vi "Broadcast Single Message.vi"(8 "error in (no error)":errorcluster, 9 "Mail Strategy In":refnum<class "Mail Strategy.lvclass">, 10 "Message In":refnum<class "Message.lvclass">, 11 "Map Tree Queue Messenger in":refnum<class "Map Tree Queue Messenger.lvclass">) -> (0 "error out":errorcluster, 3 "Map Tree Queue Messenger out":refnum<class "Map Tree Queue Messenger.lvclass">)   [LabVIEW 2024, in "Map Tree Queue Messenger.lvclass"]
uses:
  Map Tree Queue Messenger.lvclass
  Ancestor Class/Message/Message.lvclass
  Ancestor Class/Messenger/Mail Strategy/Mail Strategy.lvclass
  Map Tree Queue Messenger.lvclass/Map Tree Queue Messenger.ctl
  Ancestor Class/Messenger/Messenger Map Composite/Messenger Map Composite.lvclass/Messenger Map Composite.ctl
  Ancestor Class/Messenger/Messenger Map Composite/Public Data/Read Child Nodes.vi
  Ancestor Class/Messenger/Messenger/Messenger.lvclass
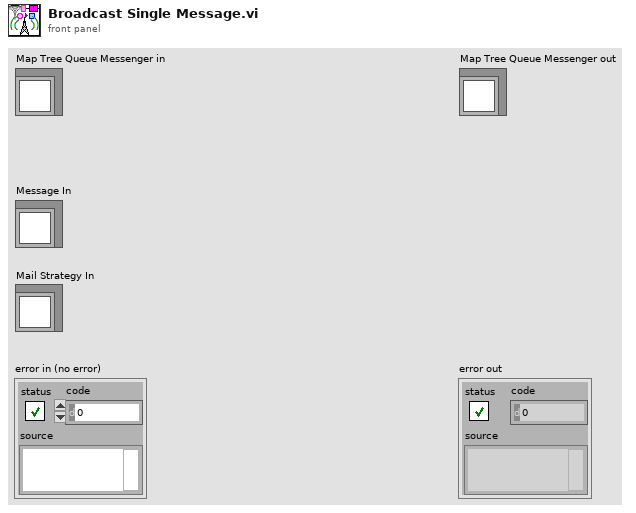
[diagram p1: front panel]
types:
  T1 = typedef "Message Queue.ctl" = refnum<queue>
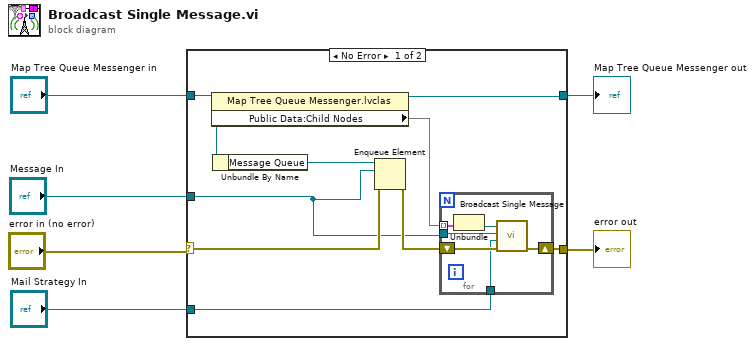
[diagram p0: block diagram]
diagram:
  n1 = case shown="No Error" "error in (no error)" {
    selector: "error in (no error)" -> [w14 w23]
    tunnel: [w12 w23] -> w2
    tunnel: [w9 w22] -> w5
    tunnel: "Map Tree Queue Messenger in" -> [w10 w22]
    tunnel: "Message In" -> [w11 _]
    tunnel: "Mail Strategy In" -> [w7 _]
    frame No Error {
      n2 = property class="Map Tree Queue Messenger.lvclas"(reference=w10) -> (reference out=w9:refnum<class "Map Tree Queue Messenger.lvclass">, "Public Data:Child Nodes"=w8:map{i64, refnum<class "Messenger.lvclass">})  [unwired: 1 in, 1 out]
      n3 = Unbundle By Name(w10) -> ("Message Queue"=w15:T1)
      n4 = Enqueue Element(queue=w15, element=w11, error in (no error)=w14) -> (error out=w13:errorcluster)  [unwired: 1 in, 2 out]
      n5 = for {
        shift-right: [w19] -> w12
        shift-left: w13 -> [w20]
        tunnel: w8 -> [w18] mode=indexing
        tunnel: w11 -> [w21]
        tunnel: w7 -> [w16]
        n6 = Unbundle(w18) -> ("Messenger"=w17:refnum<class "Messenger.lvclass">)  [unwired: 1 out]
        n7 = call-dynamic "Broadcast Single Message.vi"("error in (no error)"=w20, "Mail Strategy In"=w16, "Message In"=w21, "Messenger in"=w17) -> ("error out"=w19:errorcluster)  [unwired: 6 in, 1 out]
      }
    }
    frame Error {
    }
  }
  "error out" <- w2
  "Map Tree Queue Messenger out" <- w5
